vi "SetTestSetID.vi"(6 "Legacy (f)?":bool, 8 "error in (no error)":errorcluster, 10 "TestSetID":u32) -> (0 "error out":errorcluster)   [LabVIEW 2011]
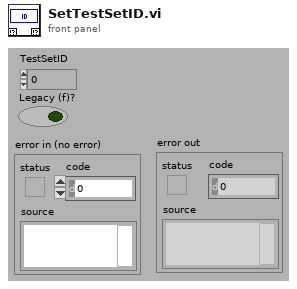
[diagram p1: front panel]
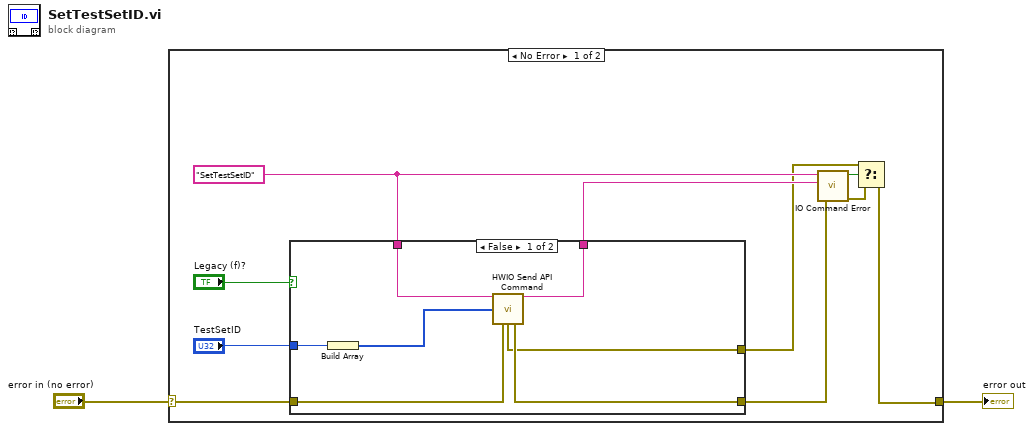
[diagram p0: block diagram]
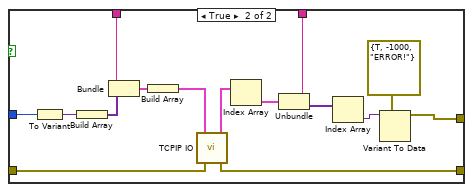
[diagram p2: hidden frame]
diagram:
  n1 = case shown="No Error" "error in (no error)" {
    selector: "error in (no error)" -> [w3 w35]
    tunnel: [w7 w35] -> w2
    frame No Error {
      w11 = "SetTestSetID"
      n2 = case shown="False" "Legacy (f)?" {
        tunnel: "TestSetID" -> [w15 w34]
        tunnel: w3 -> [w19 w31]
        tunnel: w11 -> [w16 w29]
        tunnel: [w18 w28] -> w10
        tunnel: [w17 w24] -> w9
        tunnel: [w13 w20] -> w5
        frame False {
          n3 = Build Array(w15) -> (w14:u32[])
          n4 = call "HWIO Send API Command.vi"("Action"=w16, "Integer"=w14, "error in (no error)"=w19) -> ("Action out"=w17:string, "HWError"=w13:errorcluster, "error out"=w18:errorcluster)  [unwired: 5 in, 5 out]
        }
        frame True {
          n5 = To Variant(anything=w34) -> (Variant=w33:variant)
          n6 = Build Array(w33) -> (w32:variant[])
          n7 = Bundle(w29, w32) -> (w30:cluster{string, variant[]})  [unwired: 1 out]
          n8 = Build Array(w30) -> (w27:cluster{string, variant[]}[])
          n9 = call "TCPIP IO.vi"("error in (no error)"=w31, "Commands"=w27) -> ("error out"=w28:errorcluster, "Responses"=w26:cluster{string, variant[]}[])  [unwired: 1 in, 3 out]
          n10 = Index Array(array=w26) -> (element=w25:cluster{string, variant[]})  [unwired: 1 in]
          n11 = Unbundle(w25) -> (w24:string, w21:variant[])
          n12 = Index Array(array=w21) -> (element=w23:variant)  [unwired: 1 in]
          n13 = Variant To Data(type=errorcluster {"status"=TRUE, "code"=-1000, "source"="ERROR!"} ("error out"), Variant=w23) -> (data=w20:errorcluster)  [unwired: 1 in, 1 out]
        }
      }
      n14 = call "IO Command Error.vi"("error in (no error)"=w10, "Command Returned (\"\")"=w9, "Command Sent (\"\")"=w11) -> ("error out"=w8:errorcluster, "HW ERR?"=w6:bool)  [unwired: 3 out]
      n15 = Select(t=w5, s=w6, f=w8) -> (s? t:f=w7:errorcluster)
    }
    frame Error {
    }
  }
  "error out" <- w2
